vi "Target temp.vi"(0 "elapsed time":dbl) -> (1 "Target temperature":i32, 2 "control":bool)   [LabVIEW 2016]
uses:
  Thermal_type.vi
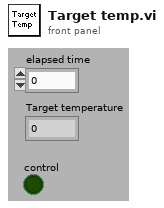
[diagram p1: front panel]
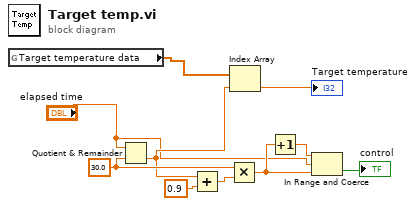
[diagram p0: block diagram]
diagram:
  w10 = 30.0 ("y")
  n1 = global read "Thermal_type.vi" "Target temperature data"() -> (w1:dbl[])
  n2 = Quotient & Remainder(x="elapsed time", y=w10) -> (floor(x/y)=w7:dbl)  [unwired: 1 out]
  n3 = Add(x=w7, y=0.9) -> (x+y=w8:dbl)
  n4 = Multiply(x=w10, y=w8) -> (x*y=w5:dbl)
  n5 = Index Array(array=w1, index=w7) -> (element=→"Target temperature":dbl)
  n6 = Increment(x=w5) -> (x+1=w6:dbl)
  n7 = In Range and Coerce(upper limit=w6, x="elapsed time", lower limit=w5) -> (In Range?=→"control":bool)  [unwired: 1 out]
